vi "Read and Update Key (Boolean).vi"(0 "Session Handle in":T1, 5 "section":string, 7 "key":string, 9 "default":bool, 11 "error in (no error)":errorcluster, 12 "create if not exists (T)":bool=TRUE) -> (4 "Session Handle out":T1, 10 "value":bool, 15 "error out":errorcluster)   [LabVIEW 2016, in "_Configurations.lvlib" / "Configurations.lvclass"]
uses:
  Configurations.lvclass
  <vilib>/Utility/config.llb/NI_LVConfig.lvlib
  <vilib>/Utility/config.llb/Write Key (Boolean).vi
  <vilib>/Utility/config.llb/Read Key (Boolean).vi
  Typedefs/Session Handle.ctl
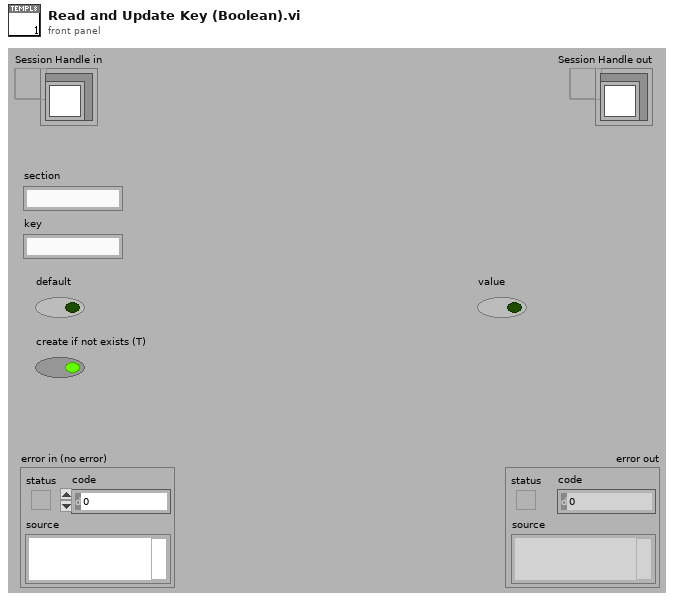
[diagram p1: front panel]
types:
  T1 = typedef "Configurations.lvlib/Configurations.lvclass/Session Handle.ctl" = refnum<data-value>
  T2 = typedef "NI_LVConfig.lvlib/Config Data RefNum.ctl" = refnum<k1>
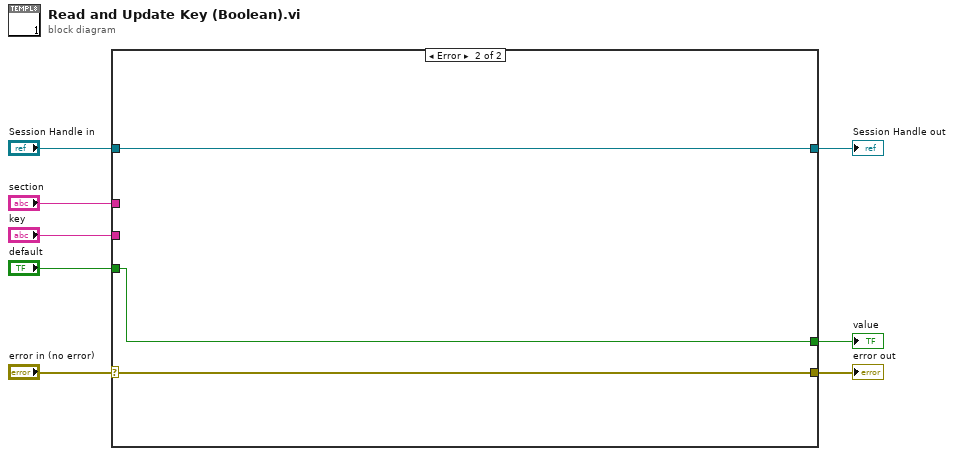
[diagram p0: block diagram]
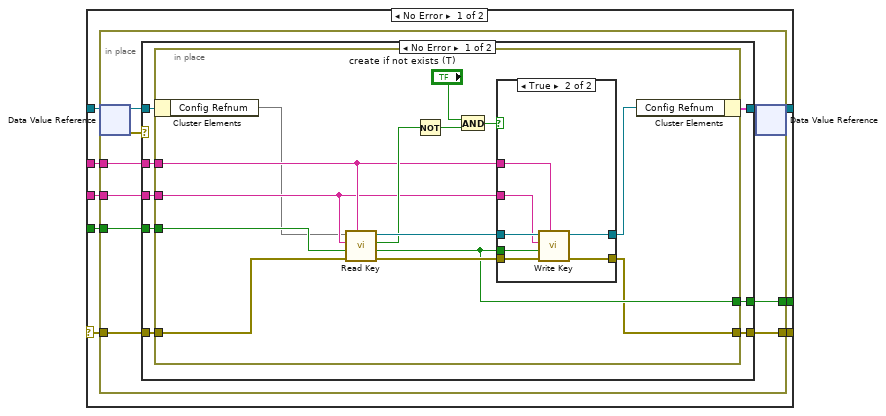
[diagram p2: hidden frame]
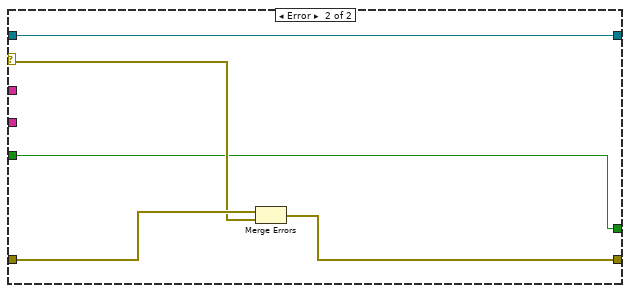
[diagram p4: hidden frame]
diagram:
  n1 = case shown="Error" "error in (no error)" {
    selector: "error in (no error)" -> [w14 w63]
    tunnel: "Session Handle in" -> [w16 w64]
    tunnel: [w15 w64] -> w7
    tunnel: [w13 w63] -> w6
    tunnel: [w12 w62] -> w4
    tunnel: "section" -> [w11 _]
    tunnel: "key" -> [w10 _]
    tunnel: "default" -> [w9 w62]
    frame No Error {
      n2 = in-place {
        in-place-border: w14 -> [w21]
        in-place-border: [w24] -> w13
        in-place-border: [w20] -> w12
        in-place-border: w11 -> [w19]
        in-place-border: w10 -> [w18]
        in-place-border: w9 -> [w17]
        n3 = in-place-dvr #1(w16) -> (w25:refnum<class "Configurations.lvclass">, w22:errorcluster)
        n4 = case shown="No Error" w22 {
          selector: w22 -> [_ w60]
          tunnel: w25 -> [w33 w58]
          tunnel: [w32 w59] -> w24
          tunnel: [w31 w58] -> w23
          tunnel: w21 -> [w30 w61]
          tunnel: [w29 w57] -> w20
          tunnel: w19 -> [w28 _]
          tunnel: w18 -> [w27 _]
          tunnel: w17 -> [w26 w57]
          frame No Error {
            n5 = in-place {
              in-place-border: [w40] -> w32
              in-place-border: w30 -> [w39]
              in-place-border: [w41] -> w29
              in-place-border: w28 -> [w38]
              in-place-border: w27 -> [w37]
              in-place-border: w26 -> [w36]
              n6 = in-place-cluster #2(w33) -> ("Config Refnum"=w35)
              n7 = call-poly <vilib>:"Read Key.vi"("section"=w38, "error in (no error)"=w39, "default value"=w36, "key"=w37, "refnum"=w35) -> ("error out"=w45:errorcluster, "value"=w41:bool, "found?"=w43:bool, "refnum out"=w44:T2)  [unwired: 3 in]
              n8 = Not(x=w43) -> (.not. x?=w46:bool)
              n9 = And(x="create if not exists (T)", y=w46) -> (x .and. y?=w42:bool)
              n10 = case shown="True" w42 {
                tunnel: w44 -> [w49 w56]
                tunnel: w45 -> [w48 w55]
                tunnel: [w48 w54] -> w40
                tunnel: [w49 w53] -> w34
                tunnel: w41 -> [_ w50]
                tunnel: w38 -> [_ w52]
                tunnel: w37 -> [_ w51]
                frame False {
                }
                frame True {
                  n11 = call-poly <vilib>:"Write Key.vi"("section"=w52, "error in (no error)"=w55, "value"=w50, "key"=w51, "refnum"=w56) -> ("error out"=w54:errorcluster, "refnum out"=w53:T2)  [unwired: 4 in, 1 out]
                }
              }
              n12 = in-place-cluster #2("Config Refnum"=w34) -> (w31:cluster{})
            }
          }
          frame Error {
            n13 = Merge Errors(w61, w60) -> (w59:errorcluster)
          }
        }
        n14 = in-place-dvr #1(w23) -> (w15:T1)  [unwired: 1 out]
      }
    }
    frame Error {
    }
  }
  "Session Handle out" <- w7
  "error out" <- w6
  "value" <- w4
